vi "Meas Sequence Loop.vi"(8 "error in":errorcluster, 11 "meas session in":T1={"adc"={"niScope"={"channel cfg"=[], "sessions"=[], "multi cards"=FALSE, "channels"=0, "type"=enum."n/a", "memory [B/chn]"=0, "ext. clock [Hz]"=0.0, "samples count"=0, "use streaming"=FALSE, "proc setup"={"packet size [smpl]"=0, "current timeout [s]"=0.0, "blk2blk timeout [s]"=0.0, "event time"=timestamp(0 s since 1904-01-01), "temp sampl T [s]"=0.0, "data queue"=refnum, "stop notifier"=refnum, "proc ref"=refnum}, "sample width [B]"=0, "ranges [V]"=[], "trigger setup"={"coupling"=1, "level [V]"=0.0, "slope"=0, "mode"=enum."Immediate"}, "fs [Hz]"=0.0, "bitres [bit]"=0}, "3458A"={"channels"=[], "sync unit"={"VISA"="", "type"=enum."Picotest U6200A"}, "awg unit"={"type"=enum."Agilent 331xxA to 332xxA", "VISA"="", "enable 10MHz ref"=FALSE}, "sync mode"=enum."MASTER-SLAVE, MASTER clocked by TIMER", "streaming mode"=FALSE, "idn mode"=enum."Auto", "sampling mode"=enum."DCV", "Ts [s]"=0.0, "sample memory [B]"=0, "proc setup"={"channel id"=0, "packet size [smpl]"=0, "current timeout [s]"=0.0, "blk2blk timeout [s]"=0.0, "event time"=timestamp(0 s since 1904-01-01), "stop notifier"=refnum, "data queues"=[], "proc refs"=[], "bus semaphore"=refnum}, "sample size [B]"=0, "sample count"=0, "aux data"={"channel id"=0, "valid?"=[], "gain [V]"=[], "timestamp [s]"=[], "Ts [s]"=0.0, "abs timestamp"=timestamp(0 s since 1904-01-01), "t [deg C]"=[]}, "ranges [V]"=[], "aperture [s]"=0.0, "LEVEL trigger"={"edge"=enum."POS", "level [V]"=0.0, "coupling"=enum."DC"}, "trigger mode"=enum."AUTO", "measure temp.?"=FALSE, "disp mesages"=[], "shared bus?"=FALSE, "disable display?"=FALSE, "aper mode"=enum."Manual", "aper rules"=[]}, "dsdll"={"dsdll"={"dsdll path"=path "", "dsdll handle"=[], "output devices"=[], "capture devices"=[]}, "channels"=0, "device id"=0, "channel idns"=[], "proc setup"={"packet size [smpl]"=0, "current timeout [s]"=0.0, "blk2blk timeout [s]"=0.0, "event time"=timestamp(0 s since 1904-01-01), "data queue"=refnum, "stop notifier"=refnum, "proc ref"=refnum}, "samples count"=0, "fs [Hz]"=0.0}, "type"=enum."niScope", "channel idn str"=[], "aux instr idn str"=[], "modified?"=FALSE, "simadc"={"channels"=[], "range [V]"=0.0, "Ts step [s]"=0.0, "time [s]"=0.0, "fs [Hz]"=0.0, "count"=0, "smpl offset"=0, "set count"=0, "bit res"=0}, "force rst?"=FALSE, "exit mode"=enum."Immediate reset", "exit dly"=0.0, "exit tmr"=timestamp(0 s since 1904-01-01), "busy?"=FALSE, "accessed?"=FALSE, "QuADC session"={"channel cfg"=[], "sessions"=[], "multi cards"=FALSE, "channels"=0, "type"=enum."n/a", "memory [B/chn]"=0, "ext. clock [Hz]"=0.0, "samples count"=0, "use streaming"=FALSE, "proc setup"={"packet size [smpl]"=0, "current timeout [s]"=0.0, "blk2blk timeout [s]"=0.0, "event time"=timestamp(0 s since 1904-01-01), "temp sampl T [s]"=0.0, "data queue"=refnum, "stop notifier"=refnum, "proc ref"=refnum}, "sample width [B]"=0, "ranges [V]"=[], "trigger setup"={"coupling"=1, "level [V]"=0.0, "slope"=0, "mode"=enum."Immediate"}, "fs [Hz]"=0.0, "bitres [bit]"=0}}, "sequence"=[], "sequence setup"={"group setups"=[], "average cycles"=0, "range mode"=enum."Keep defaults", "fs mode"=enum."Frequency", "rng even"=0.0, "rng odd"=0.0, "folder"=path "", "name base"="", "meas id"=0, "settle [s]"=0.0}, "golpi"=refnum, "processing setup"={"mode"=enum."Raw", "call after avgs?"=FALSE, "calculate?"=FALSE, "raw mode"={"command"="", "result mode"=enum."Display console output (only Octave)", "res variable"=""}, "QWTB"={"QWTB path"=path "", "alg filter path"="", "alg ids"=[], "alg parameters"=[], "parsed parameters"=[], "selected alg id"="", "selected unc mode"=enum."None", "qwtb mcc"=100, "qwtb timeout"=90, "qwtb covg"=95.0, "qwtb ofs"=0, "qwtb lim data"=0, "multicore"={"jobs folder"=path "", "cores"=0, "max jobs"=0, "mode"=enum."Singlecore"}, "unc once?"=FALSE}}, "corrections"={"transducers"={"channels"=[], "last path"=path ""}, "digitizer"={"last path"=path "", "channel paths"=[], "channel idns"=[], "correction name"="", "channel names"=[], "folders to copy"=[], "channel valid"=[], "correction path"=path "", "correction rel path"="", "rel folders to copy"=[]}}, "assist cfg"={"P"=0, "Q"=0, "rel shift"=0.0, "ref freq"=0.0, "min fs"=0.0, "max fs tol"=0.0, "min int"=0.0, "max int"=0.0, "max err"=0.0, "max timeout"=0.0}} {"corrections"."transducers"."channels"."Phase index" min=1 step=1; "adc"."QuADC session"."trigger setup"."level [V]" format="%.2f"; "adc"."QuADC session"."trigger setup"."coupling" items=["AC"=0, "DC"=1, "HF Reject"=3, "LF Reject"=4, "AC Plus HF Reject"=1001]; "adc"."QuADC session"."channel cfg"."Clock fr. (Hz)" min=0.0 format="%#_9p"; "adc"."QuADC session"."channel cfg"."Number of JJ" min=1; "adc"."QuADC session"."channel cfg"."Range [Vpk]" min=0.0; "adc"."QuADC session"."channel cfg"."Channel" min=0; "adc"."3458A"."channels"."Range [Vpk]" min=0.0; "adc"."niScope"."trigger setup"."level [V]" format="%.2f"; "adc"."niScope"."trigger setup"."coupling" items=["AC"=0, "DC"=1, "HF Reject"=3, "LF Reject"=4, "AC Plus HF Reject"=1001]; "adc"."niScope"."channel cfg"."Range [Vpk]" min=0.0; "adc"."niScope"."channel cfg"."Channel" min=0}) -> (0 "error out":errorcluster, 3 "meas session out":T1={"adc"={"niScope"={"channel cfg"=[], "sessions"=[], "multi cards"=FALSE, "channels"=0, "type"=enum."n/a", "memory [B/chn]"=0, "ext. clock [Hz]"=0.0, "samples count"=0, "use streaming"=FALSE, "proc setup"={"packet size [smpl]"=0, "current timeout [s]"=0.0, "blk2blk timeout [s]"=0.0, "event time"=timestamp(0 s since 1904-01-01), "temp sampl T [s]"=0.0, "data queue"=refnum, "stop notifier"=refnum, "proc ref"=refnum}, "sample width [B]"=0, "ranges [V]"=[], "trigger setup"={"coupling"=1, "level [V]"=0.0, "slope"=0, "mode"=enum."Immediate"}, "fs [Hz]"=0.0, "bitres [bit]"=0}, "3458A"={"channels"=[], "sync unit"={"VISA"="", "type"=enum."Picotest U6200A"}, "awg unit"={"type"=enum."Agilent 331xxA to 332xxA", "VISA"="", "enable 10MHz ref"=FALSE}, "sync mode"=enum."MASTER-SLAVE, MASTER clocked by TIMER", "streaming mode"=FALSE, "idn mode"=enum."Auto", "sampling mode"=enum."DCV", "Ts [s]"=0.0, "sample memory [B]"=0, "proc setup"={"channel id"=0, "packet size [smpl]"=0, "current timeout [s]"=0.0, "blk2blk timeout [s]"=0.0, "event time"=timestamp(0 s since 1904-01-01), "stop notifier"=refnum, "data queues"=[], "proc refs"=[], "bus semaphore"=refnum}, "sample size [B]"=0, "sample count"=0, "aux data"={"channel id"=0, "valid?"=[], "gain [V]"=[], "timestamp [s]"=[], "Ts [s]"=0.0, "abs timestamp"=timestamp(0 s since 1904-01-01), "t [deg C]"=[]}, "ranges [V]"=[], "aperture [s]"=0.0, "LEVEL trigger"={"edge"=enum."POS", "level [V]"=0.0, "coupling"=enum."DC"}, "trigger mode"=enum."AUTO", "measure temp.?"=FALSE, "disp mesages"=[], "shared bus?"=FALSE, "disable display?"=FALSE, "aper mode"=enum."Manual", "aper rules"=[]}, "dsdll"={"dsdll"={"dsdll path"=path "", "dsdll handle"=[], "output devices"=[], "capture devices"=[]}, "channels"=0, "device id"=0, "channel idns"=[], "proc setup"={"packet size [smpl]"=0, "current timeout [s]"=0.0, "blk2blk timeout [s]"=0.0, "event time"=timestamp(0 s since 1904-01-01), "data queue"=refnum, "stop notifier"=refnum, "proc ref"=refnum}, "samples count"=0, "fs [Hz]"=0.0}, "type"=enum."niScope", "channel idn str"=[], "aux instr idn str"=[], "modified?"=FALSE, "simadc"={"channels"=[], "range [V]"=0.0, "Ts step [s]"=0.0, "time [s]"=0.0, "fs [Hz]"=0.0, "count"=0, "smpl offset"=0, "set count"=0, "bit res"=0}, "force rst?"=FALSE, "exit mode"=enum."Immediate reset", "exit dly"=0.0, "exit tmr"=timestamp(0 s since 1904-01-01), "busy?"=FALSE, "accessed?"=FALSE, "QuADC session"={"channel cfg"=[], "sessions"=[], "multi cards"=FALSE, "channels"=0, "type"=enum."n/a", "memory [B/chn]"=0, "ext. clock [Hz]"=0.0, "samples count"=0, "use streaming"=FALSE, "proc setup"={"packet size [smpl]"=0, "current timeout [s]"=0.0, "blk2blk timeout [s]"=0.0, "event time"=timestamp(0 s since 1904-01-01), "temp sampl T [s]"=0.0, "data queue"=refnum, "stop notifier"=refnum, "proc ref"=refnum}, "sample width [B]"=0, "ranges [V]"=[], "trigger setup"={"coupling"=1, "level [V]"=0.0, "slope"=0, "mode"=enum."Immediate"}, "fs [Hz]"=0.0, "bitres [bit]"=0}}, "sequence"=[], "sequence setup"={"group setups"=[], "average cycles"=0, "range mode"=enum."Keep defaults", "fs mode"=enum."Frequency", "rng even"=0.0, "rng odd"=0.0, "folder"=path "", "name base"="", "meas id"=0, "settle [s]"=0.0}, "golpi"=refnum, "processing setup"={"mode"=enum."Raw", "call after avgs?"=FALSE, "calculate?"=FALSE, "raw mode"={"command"="", "result mode"=enum."Display console output (only Octave)", "res variable"=""}, "QWTB"={"QWTB path"=path "", "alg filter path"="", "alg ids"=[], "alg parameters"=[], "parsed parameters"=[], "selected alg id"="", "selected unc mode"=enum."None", "qwtb mcc"=100, "qwtb timeout"=90, "qwtb covg"=95.0, "qwtb ofs"=0, "qwtb lim data"=0, "multicore"={"jobs folder"=path "", "cores"=0, "max jobs"=0, "mode"=enum."Singlecore"}, "unc once?"=FALSE}}, "corrections"={"transducers"={"channels"=[], "last path"=path ""}, "digitizer"={"last path"=path "", "channel paths"=[], "channel idns"=[], "correction name"="", "channel names"=[], "folders to copy"=[], "channel valid"=[], "correction path"=path "", "correction rel path"="", "rel folders to copy"=[]}}, "assist cfg"={"P"=0, "Q"=0, "rel shift"=0.0, "ref freq"=0.0, "min fs"=0.0, "max fs tol"=0.0, "min int"=0.0, "max int"=0.0, "max err"=0.0, "max timeout"=0.0}} {"corrections"."transducers"."channels"."Phase index" min=1 step=1; "adc"."QuADC session"."trigger setup"."level [V]" format="%.2f"; "adc"."QuADC session"."trigger setup"."coupling" items=["AC"=0, "DC"=1, "HF Reject"=3, "LF Reject"=4, "AC Plus HF Reject"=1001]; "adc"."QuADC session"."channel cfg"."Clock fr. (Hz)" min=0.0 format="%#_9p"; "adc"."QuADC session"."channel cfg"."Number of JJ" min=1; "adc"."QuADC session"."channel cfg"."Range [Vpk]" min=0.0; "adc"."QuADC session"."channel cfg"."Channel" min=0; "adc"."3458A"."channels"."Range [Vpk]" min=0.0; "adc"."niScope"."trigger setup"."level [V]" format="%.2f"; "adc"."niScope"."trigger setup"."coupling" items=["AC"=0, "DC"=1, "HF Reject"=3, "LF Reject"=4, "AC Plus HF Reject"=1001]; "adc"."niScope"."channel cfg"."Range [Vpk]" min=0.0; "adc"."niScope"."channel cfg"."Channel" min=0})   [LabVIEW 2013]
doc: "This VI initiates sampling of one record with current setup of ADC. It streams the sample data to MAT file of a given path (without extension). The VI also appends logged temperatures to the MAT file. It will return ADC auxiliary data which are valid only if flag 'valid?' in the cluster is True (that should happen all the time except when the sampling was aborted for whatever reason). The VI responds to global stop button called 'btn stop' - it will abort sampling when it is in True state."
uses:
  Meas Session.ctl
  adc/ADC Session.ctl
  drivers/niScope/niScope Session.ctl
  drivers/niScope/niScope Virtual Channel Config.ctl
  drivers/niScope/niScope Virtual Channel Mode.ctl
  drivers/niScope/niScope Virtual Channel Input Z.ctl
  drivers/niScope/niScope Virtual Channel Coupling.ctl
  drivers/niScope/niScope Type.ctl
  drivers/niScope/niScope Digitizing Process Options.ctl
  drivers/niScope/niScope Data Packet.ctl
  drivers/niScope/niScope Trigger Setup.ctl
  <instrlib>/niScope/Controls/niScope trigger coupling.ctl
  <instrlib>/niScope/Controls/niScope trigger slope.ctl
  drivers/DMM/3458A Digitizer Session.ctl
  drivers/DMM/3458A Virtual Channel Config.ctl
  drivers/Counter/Counter Session.ctl
  drivers/Counter/Counter Type.ctl
  drivers/AWG/AWG Session.ctl
  drivers/AWG/AWG Type.ctl
  drivers/DMM/3458A Sync Mode.ctl
  drivers/DMM/3458A Idn Mode.ctl
  drivers/DMM/3458A Digitizing Low Levels/Configure/Sampling Mode.ctl
  drivers/DMM/3458A Digitizing Process Options.ctl
  drivers/DMM/3458A Data Packet.ctl
  drivers/DMM/3458A Aux Record Data.ctl
  drivers/DMM/3458A Digitizing Low Levels/Configure/Level Setup.ctl
  drivers/DMM/3458A Digitizing Low Levels/Configure/First Sample Trigger.ctl
  drivers/DMM/3458A Aperture Selection Mode.ctl
  drivers/dsdll/DSDLL Session.ctl
  drivers/dsdll/dsdll.lvlibp/dsdll_instance.ctl
  drivers/dsdll/dsdll.lvlibp/dsdll_device_record.ctl
  drivers/dsdll/DSDLL Process Config.ctl
  drivers/dsdll/DSDLL Data Packet.ctl
  adc/ADC Type.ctl
  drivers/simulated_adc/SimAdc Config.ctl
  drivers/simulated_adc/SimAdc Channel Cfg.ctl
  adc/ADC On Close Action.ctl
  drivers/Quatsch_driver/QuADCDriver/QuADC Session.ctl
  drivers/Quatsch_driver/QuADCDriver/QuADC Virtual Channel Config.ctl
  drivers/Quatsch_driver/QuADCDriver/QuADC Virtual Channel Mode.ctl
  drivers/Quatsch_driver/QuADCDriver/QuADC Virtual Channel Input Z.ctl
  drivers/Quatsch_driver/QuADCDriver/QuADC Virtual Channel Coupling.ctl
  drivers/Quatsch_driver/QuADCDriver/QuADC Type.ctl
  drivers/Quatsch_driver/QuADCDriver/QuADC Digitizing Process Options.ctl
  drivers/Quatsch_driver/QuADCDriver/QuADC Data Packet.ctl
  drivers/Quatsch_driver/QuADCDriver/QuADC Trigger Setup.ctl
  Meas Sequence Item.ctl
  Meas Sampling Configuration.ctl
  adc/ADC Trig Config.ctl
  adc/ADC Trig Mode Source.ctl
  adc/ADC Trig Coupling.ctl
  adc/ADC Trig Slope.ctl
  processing/QWTB/Meas Proc QWTB Algorithm Parameter Data.ctl
  Meas Sequence Configuration.ctl
  Meas Range Mode.ctl
  Meas Sampling Rate Mode.ctl
  octave/golpi/mpc/golpi_session_ref.ctl
  octave/golpi/mpc/golpi_session.ctl
  octave/golpi/GOLPI Library.lvlibp/Public/GOLPI reference Type Def.ctl
  octave/golpi/GOLPI Library.lvlibp/LV Process source distribution/Pipe Handle.ctl
  processing/Meas Process Config.ctl
  processing/Meas Process Mode.ctl
  processing/Meas Process Raw Config.ctl
  processing/Meas Process Raw Result Mode.ctl
  processing/QWTB/Meas Proc QWTB Setup.ctl
  processing/QWTB/Meas Proc QWTB Uncertainty Mode.ctl
  processing/QWTB/Meas Proc QWTB Multicore Setup.ctl
  processing/QWTB/Meas Proc QWTB Multicore Type.ctl
  Corrections/Corr Setup.ctl
  Corrections/Corr Tranducer Item.ctl
  Corrections/Corr Digitizers.ctl
  Assist/Assist Panel Setup.ctl
  varilib/SGUI Assign Multiple Strings With Tags By Label.vi
  varilib/varilib.lvlib
  drivers/niScope/niScope Virtual Digitizer.lvlib
  drivers/DMM/3458A Virtual Digitizer.lvlib
  drivers/Counter/Counter.lvlib
  drivers/AWG/AWG.lvlib
  drivers/DMM/3458A Digitizing Low Levels/3458A Digitizing Low Levels.lvlib
  drivers/dsdll/dsdll.lvlibp
  drivers/dsdll/DSDLL Virtual Digitizer.lvlib
  octave/golpi/GOLPI Library.lvlibp/LV Process source distribution/LV Process library.lvlib
  octave/golpi/GOLPI Library.lvlibp
  octave/golpi/mpc/GOLPI Multi Process.lvlib
  drivers/Quatsch_driver/QuADCDriver/QuADC Virtual Digitizer.lvlib
panel:
  # "ADC:"
  # "IP Address"
  # "."
  # "."
  # "."
  # ":"
  # "ADC:"
  # "IP Address"
  # "."
  # "."
  # "."
  # ":"
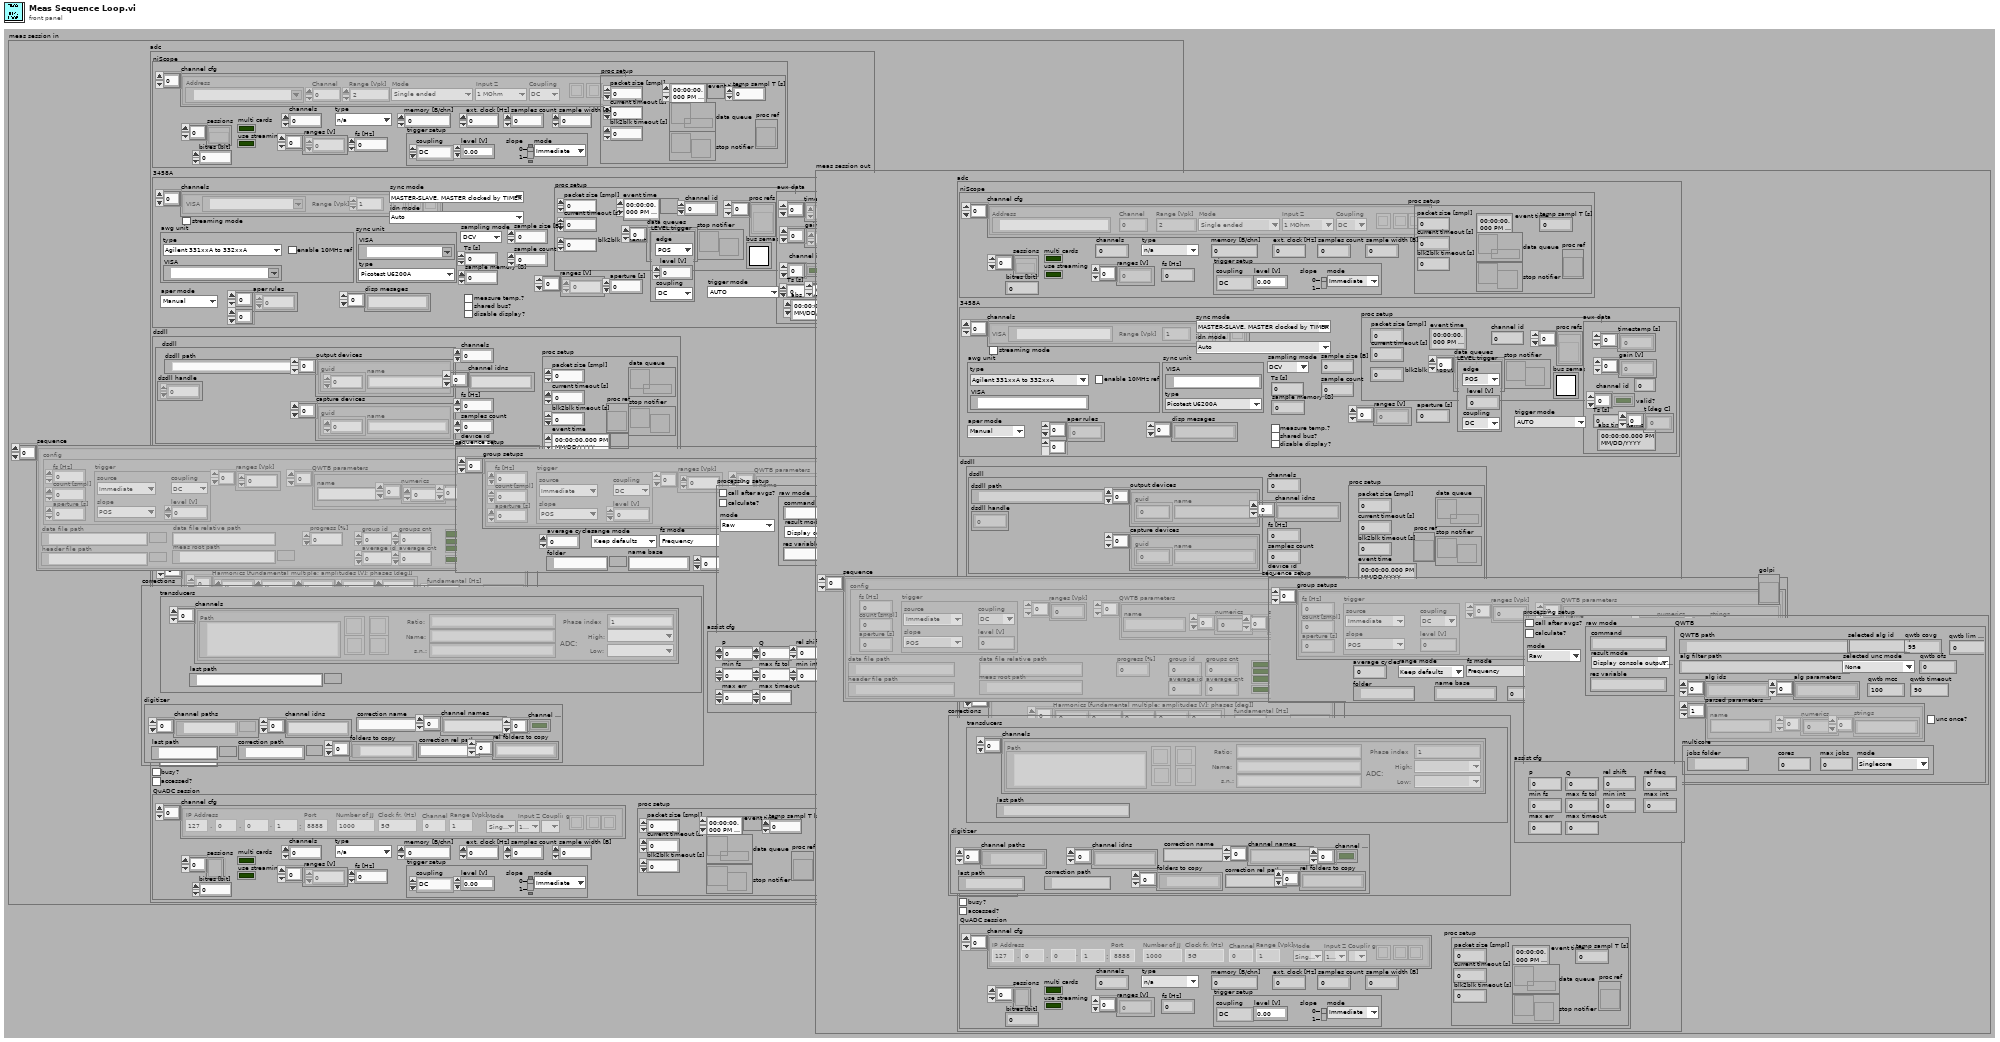
[diagram p1: front panel]
types:
  T1 = typedef "Meas Session.ctl" = cluster{"adc":T2, "sequence":T44[], "sequence setup":T51, "golpi":T54, "processing setup":T55, "corrections":T63, "assist cfg":T66}
  T2 = typedef "ADC Session.ctl" = cluster{"niScope":T3, "3458A":T13, "dsdll":T28, "type":T32, "channel idn str":string[], "aux instr idn str":string[], "modified?":bool, "simadc":T33, "force rst?":bool, "exit mode":T35, "exit dly":dbl, "exit tmr":timestamp, "busy?":bool, "accessed?":bool, "QuADC session":T36}
  T3 = typedef "niScope Virtual Digitizer.lvlib/niScope Session.ctl" = cluster{"channel cfg":T4[], "sessions":refnum<k20>[], "multi cards":bool, "channels":i32, "type":T8, "memory [B/chn]":i32, "ext. clock [Hz]":dbl, "samples count":i64, "use streaming":bool, "proc setup":T9, "sample width [B]":i32, "ranges [V]":dbl[], "trigger setup":T10, "fs [Hz]":dbl, "bitres [bit]":i32}
  T4 = typedef "niScope Virtual Digitizer.lvlib/niScope Virtual Channel Config.ctl" = cluster{"Address":refnum<k15>, "Channel":i32, "Mode":T5, "Input Z":T6, "Coupling":T7, "Range [Vpk]":dbl, "btn clr":bool, "btn up":bool, "btn down":bool}
  T5 = typedef "niScope Virtual Digitizer.lvlib/niScope Virtual Channel Mode.ctl" = enum16{"Single ended", "Unbal. differential", "Differential"}
  T6 = typedef "niScope Virtual Digitizer.lvlib/niScope Virtual Channel Input Z.ctl" = enum16{"1 MOhm", "50 Ohm"}
  T7 = typedef "niScope Virtual Digitizer.lvlib/niScope Virtual Channel Coupling.ctl" = enum16{"AC", "DC", "GND"}
  T8 = typedef "niScope Virtual Digitizer.lvlib/niScope Type.ctl" = enum16{"n/a", "5922"}
  T9 = typedef "niScope Virtual Digitizer.lvlib/niScope Digitizing Process Options.ctl" = cluster{"packet size [smpl]":i64, "current timeout [s]":dbl, "blk2blk timeout [s]":dbl, "event time":timestamp, "temp sampl T [s]":dbl, "data queue":refnum<queue>, "stop notifier":refnum<notifier>, "proc ref":refnum<vi>}
  T10 = typedef "niScope Virtual Digitizer.lvlib/niScope Trigger Setup.ctl" = cluster{"coupling":T11, "level [V]":dbl, "slope":T12, "mode":enum16{"Immediate", "External", "Level"}}
  T11 = typedef "niScope trigger coupling.ctl" = u16
  T12 = typedef "niScope trigger slope.ctl" = i32
  T13 = typedef "3458A Virtual Digitizer.lvlib/3458A Digitizer Session.ctl" = cluster{"channels":T14[], "sync unit":T15, "awg unit":T17, "sync mode":T19, "streaming mode":bool, "idn mode":T20, "sampling mode":T21, "Ts [s]":dbl, "sample memory [B]":i32, "proc setup":T22, "sample size [B]":i32, "sample count":i32, "aux data":T24, "ranges [V]":dbl[], "aperture [s]":dbl, "LEVEL trigger":T25, "trigger mode":T26, "measure temp.?":bool, "disp mesages":string[], "shared bus?":bool, "disable display?":bool, "aper mode":T27, "aper rules":dbl[][]}
  T14 = typedef "3458A Virtual Digitizer.lvlib/3458A Virtual Channel Config.ctl" = cluster{"VISA":refnum<visa-resource-name>, "Range [Vpk]":dbl, "btn clr":bool, "btn up":bool, "btn down":bool}
  T15 = typedef "Counter.lvlib/Counter Session.ctl" = cluster{"VISA":refnum<visa-resource-name>, "type":T16}
  T16 = typedef "Counter.lvlib/Counter Type.ctl" = enum16{"Picotest U6200A", "dummy"}
  T17 = typedef "AWG.lvlib/AWG Session.ctl" = cluster{"type":T18, "VISA":refnum<visa-resource-name>, "enable 10MHz ref":bool}
  T18 = typedef "AWG.lvlib/AWG Type.ctl" = enum16{"Agilent 331xxA to 332xxA", "Agilent 335xxA to 336xxA", "Tektronix AFG3101C", "dummy"}
  T19 = typedef "3458A Virtual Digitizer.lvlib/3458A Sync Mode.ctl" = enum16{"MASTER-SLAVE, MASTER clocked by TIMER", "MASTER-SLAVE, MASTER clocked by AWG", "ALL clocked by AWG", "MASTER-SLAVE, ALL clocked by TIMER", "ALL clocked by AWG with DFLL"}
  T20 = typedef "3458A Virtual Digitizer.lvlib/3458A Idn Mode.ctl" = enum16{"Auto", "Sequential (chn A, chn B, ...)", "From calibration string"}
  T21 = typedef "3458A Virtual Digitizer.lvlib/3458A Digitizing Low Levels.lvlib/Sampling Mode.ctl" = enum16{"DCV", "DSDC", "DSAC"}
  T22 = typedef "3458A Virtual Digitizer.lvlib/3458A Digitizing Process Options.ctl" = cluster{"channel id":i32, "packet size [smpl]":i32, "current timeout [s]":dbl, "blk2blk timeout [s]":dbl, "event time":timestamp, "stop notifier":refnum<notifier>, "data queues":refnum<queue>[], "proc refs":refnum<vi>[], "bus semaphore":T23}
  T23 = typedef "Semaphore RefNum" = refnum<k1>
  T24 = typedef "3458A Virtual Digitizer.lvlib/3458A Aux Record Data.ctl" = cluster{"channel id":i32, "valid?":bool[], "gain [V]":dbl[], "timestamp [s]":dbl[], "Ts [s]":dbl, "abs timestamp":timestamp, "t [deg C]":dbl[]}
  T25 = typedef "3458A Virtual Digitizer.lvlib/3458A Digitizing Low Levels.lvlib/Level Setup.ctl" = cluster{"edge":enum16{"POS", "NEG"}, "level [V]":dbl, "coupling":enum16{"DC", "AC"}}
  T26 = typedef "3458A Virtual Digitizer.lvlib/3458A Digitizing Low Levels.lvlib/First Sample Trigger.ctl" = enum16{"AUTO", "EXT", "SYN", "SGL", "HOLD", "LEVEL"}
  T27 = typedef "3458A Virtual Digitizer.lvlib/3458A Aperture Selection Mode.ctl" = enum16{"Manual", "Maximum", "Table"}
  T28 = typedef "DSDLL Virtual Digitizer.lvlib/DSDLL Session.ctl" = cluster{"dsdll":T29, "channels":i32, "device id":i32, "channel idns":string[], "proc setup":T31, "samples count":i32, "fs [Hz]":dbl}
  T29 = typedef "dsdll.lvlibp/dsdll_instance.ctl" = cluster{"dsdll path":path, "dsdll handle":u8[], "output devices":T30[], "capture devices":T30[]}
  T30 = typedef "dsdll.lvlibp/dsdll_device_record.ctl" = cluster{"guid":u8[], "name":string}
  T31 = typedef "DSDLL Virtual Digitizer.lvlib/DSDLL Process Config.ctl" = cluster{"packet size [smpl]":i32, "current timeout [s]":dbl, "blk2blk timeout [s]":dbl, "event time":timestamp, "data queue":refnum<queue>, "stop notifier":refnum<notifier>, "proc ref":refnum<vi>}
  T32 = typedef "ADC Type.ctl" = enum16{"niScope", "3458A", "DirectSound DLL", "dummy", "QuADC"}
  T33 = typedef "SimAdc Config.ctl" = cluster{"channels":T34[], "range [V]":dbl, "Ts step [s]":dbl, "time [s]":dbl, "fs [Hz]":dbl, "count":i64, "smpl offset":i64, "set count":i64, "bit res":i32}
  T34 = typedef "SimAdc Channel Cfg.ctl" = cluster{"harmonics":dbl[][], "btn clear":bool, "noise":dbl, "fundamental [Hz]":dbl}
  T35 = typedef "ADC On Close Action.ctl" = enum16{"Immediate reset", "Delayed reset"}
  T36 = typedef "QuADC Virtual Digitizer.lvlib/QuADC Session.ctl" = cluster{"channel cfg":T37[], "sessions":refnum<k5>[], "multi cards":bool, "channels":i32, "type":T41, "memory [B/chn]":i32, "ext. clock [Hz]":dbl, "samples count":i64, "use streaming":bool, "proc setup":T42, "sample width [B]":i32, "ranges [V]":dbl[], "trigger setup":T43, "fs [Hz]":dbl, "bitres [bit]":i32}
  T37 = typedef "QuADC Virtual Digitizer.lvlib/QuADC Virtual Channel Config.ctl" = cluster{"Channel":i32, "Mode":T38, "Input Z":T39, "Coupling":T40, "Range [Vpk]":dbl, "btn clr":bool, "btn up":bool, "btn down":bool, "IP address A":u8, "IP address B":u8, "IP address C":u8, "IP address D":u8, "Port":u16, "Number of JJ":u32, "Clock fr. (Hz)":dbl}
  T38 = typedef "QuADC Virtual Digitizer.lvlib/QuADC Virtual Channel Mode.ctl" = enum16{"Single ended", "Unbal. differential", "Differential"}
  T39 = typedef "QuADC Virtual Digitizer.lvlib/QuADC Virtual Channel Input Z.ctl" = enum16{"1 MOhm", "50 Ohm"}
  T40 = typedef "QuADC Virtual Digitizer.lvlib/QuADC Virtual Channel Coupling.ctl" = enum16{"AC", "DC", "GND"}
  T41 = typedef "QuADC Virtual Digitizer.lvlib/QuADC Type.ctl" = enum16{"n/a", "v1"}
  T42 = typedef "QuADC Virtual Digitizer.lvlib/QuADC Digitizing Process Options.ctl" = cluster{"packet size [smpl]":i64, "current timeout [s]":dbl, "blk2blk timeout [s]":dbl, "event time":timestamp, "temp sampl T [s]":dbl, "data queue":refnum<queue>, "stop notifier":refnum<notifier>, "proc ref":refnum<vi>}
  T43 = typedef "QuADC Virtual Digitizer.lvlib/QuADC Trigger Setup.ctl" = cluster{"coupling":T11, "level [V]":dbl, "slope":T12, "mode":enum16{"Immediate", "External", "Level"}}
  T44 = typedef "Meas Sequence Item.ctl" = cluster{"config":T45, "data file path":path, "header file path":path, "group id":i32, "average id":i32, "group done?":bool, "adc modified?":bool, "source modified?":bool, "progress [%]":dbl, "groups cnt":i32, "average cnt":i32, "data file relative path":string, "meas root path":path, "calculate?":bool}
  T45 = typedef "Meas Sampling Configuration.ctl" = cluster{"fs [Hz]":dbl, "count [smpl]":i64, "aperture [s]":dbl, "trigger":T46, "ranges [Vpk]":dbl[], "QWTB parameters":T50[]}
  T46 = typedef "ADC Trig Config.ctl" = cluster{"source":T47, "level [V]":dbl, "coupling":T48, "slope":T49}
  T47 = typedef "ADC Trig Mode Source.ctl" = enum16{"Immediate", "External", "Level"}
  T48 = typedef "ADC Trig Coupling.ctl" = enum16{"DC", "AC"}
  T49 = typedef "ADC Trig Slope.ctl" = enum16{"POS", "NEG"}
  T50 = typedef "Meas Proc QWTB Algorithm Parameter Data.ctl" = cluster{"name":string, "numerics":dbl[], "strings":string[]}
  T51 = typedef "Meas Sequence Configuration.ctl" = cluster{"group setups":T45[], "average cycles":i32, "range mode":T52, "fs mode":T53, "rng even":dbl, "rng odd":dbl, "folder":path, "name base":string, "meas id":i32, "settle [s]":dbl}
  T52 = typedef "Meas Range Mode.ctl" = enum16{"Keep defaults", "Set All channels", "Set Odd and Even channels"}
  T53 = typedef "Meas Sampling Rate Mode.ctl" = enum16{"Frequency", "Period"}
  T54 = typedef "GOLPI Multi Process.lvlib/golpi_session_ref.ctl" = refnum<vi>
  T55 = typedef "Meas Process Config.ctl" = cluster{"mode":T56, "call after avgs?":bool, "calculate?":bool, "raw mode":T57, "QWTB":T59}
  T56 = typedef "Meas Process Mode.ctl" = enum16{"Raw", "QWTB"}
  T57 = typedef "Meas Process Raw Config.ctl" = cluster{"command":string, "result mode":T58, "res variable":string}
  T58 = typedef "Meas Process Raw Result Mode.ctl" = enum16{"Display console output (only Octave)", "Display string variable", "Display result file %respath%"}
  T59 = typedef "Meas Proc QWTB Setup.ctl" = cluster{"QWTB path":path, "alg filter path":string, "alg ids":string[], "alg parameters":string[], "parsed parameters":T50[], "selected alg id":string, "selected unc mode":T60, "qwtb mcc":i32, "qwtb timeout":i32, "qwtb covg":dbl, "qwtb ofs":i64, "qwtb lim data":i64, "multicore":T61, "unc once?":bool}
  T60 = typedef "Meas Proc QWTB Uncertainty Mode.ctl" = enum16{"None", "GUF", "Monte Carlo"}
  T61 = typedef "Meas Proc QWTB Multicore Setup.ctl" = cluster{"jobs folder":path, "cores":i32, "max jobs":i32, "mode":T62}
  T62 = typedef "Meas Proc QWTB Multicore Type.ctl" = enum16{"Singlecore", "Multicore", "Multistation"}
  T63 = typedef "Corr Setup.ctl" = cluster{"transducers":cluster{"channels":T64[], "last path":path}, "digitizer":T65}
  T64 = typedef "Corr Tranducer Item.ctl" = cluster{"Path":path, "Ratio:":string, "Name:":string, "btn rem":bool, "btn up":bool, "btn down":bool, "s.n.:":string, "btn open":bool, "ratio o/i":dbl, "chn hi":u16, "chn lo":u16, "Phase index":i32}
  T65 = typedef "Corr Digitizers.ctl" = cluster{"last path":path, "channel paths":path[], "channel idns":string[], "correction name":string, "channel names":string[], "folders to copy":path[], "channel valid":bool[], "correction path":path, "correction rel path":string, "rel folders to copy":string[]}
  T66 = typedef "Assist Panel Setup.ctl" = cluster{"P":i32, "Q":i32, "rel shift":dbl, "ref freq":dbl, "min fs":dbl, "max fs tol":dbl, "min int":dbl, "max int":dbl, "max err":dbl, "max timeout":dbl}
  T67 = typedef "ADC Aux Data.ctl" = cluster{"offset [V]":dbl[], "gain [V]":dbl[], "time stamp [s]":dbl[], "increment [s]":dbl, "T smpl":i64[], "T [deg C]":dbl[][], "valid?":bool, "abs timestamp":timestamp}
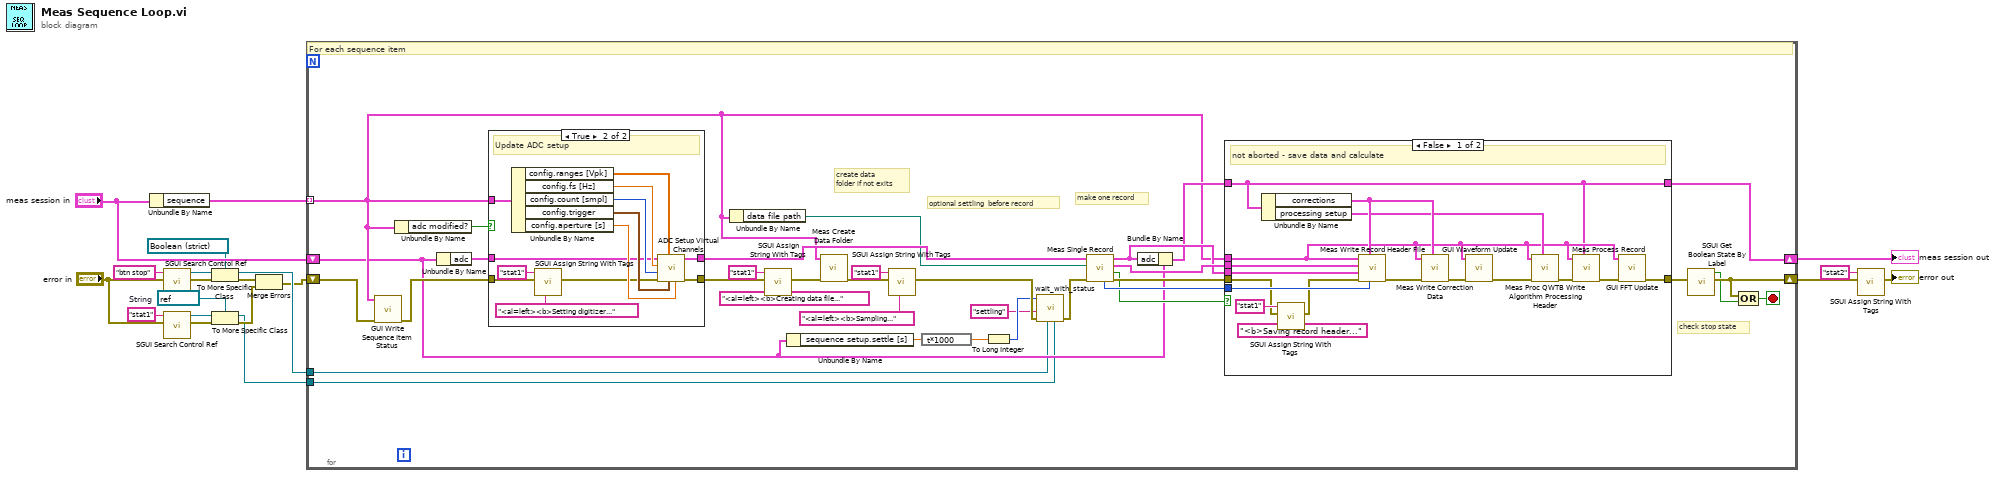
[diagram p0: block diagram]
diagram:
  w3 = refnum<vi> refnum  # String
  n1 = Unbundle By Name("meas session in") -> ("sequence"=w19:T44[])
  n2 = call "SGUI Search Control Ref.vi"("error in"="error in", "control label (empty)"="btn stop") -> ("error out"=w13:errorcluster, "control ref out"=w11:refnum<vi>)  [unwired: 7 in, 1 out]
  n3 = call "SGUI Search Control Ref.vi"("error in"="error in", "control label (empty)"="stat1") -> ("error out"=w9:errorcluster, "control ref out"=w5:refnum<vi>)  [unwired: 7 in, 1 out]
  n4 = To More Specific Class(target class=refnum<vi> refnum ("Boolean"), reference=w11, error in=w13) -> (specific class reference=w12:refnum<vi>, error out=w8:errorcluster)
  n5 = To More Specific Class(target class=w3, reference=w5, error in=w9) -> (specific class reference=w4:refnum<vi>, error out=w7:errorcluster)
  n6 = Merge Errors(w8, w7) -> (w6:errorcluster)
  n7 = for {
    tunnel: w19 -> [w31] mode=indexing
    shift-right: [w45] -> w18
    shift-left: w6 -> [w30]
    shift-right: [w32] -> w20
    shift-left: "meas session in" -> [w27]
    tunnel: w12 -> [w23]
    tunnel: w4 -> [w22]
    stop <- w46 stop-if-true
    # "optional settling  before record"
    # "create data\nfolder if not exits"
    # "check stop state"
    # "make one record"
    # "For each sequence item"
    n8 = call "GUI Write Sequence Item Status.vi"("error in"=w30, "sequence item"=w31) -> ("error out"=w35:errorcluster)  [unwired: 8 in, 1 out]
    n9 = Unbundle By Name(w31) -> ("adc modified?"=w53:bool)
    n10 = Unbundle By Name(w27) -> ("adc"=w54:T2)
    n11 = case shown="True" w53 {
      tunnel: w35 -> [w74 w79]
      tunnel: w31 -> [_ w83]
      tunnel: w54 -> [w75 w82]
      tunnel: [w74 w81] -> w42
      tunnel: [w75 w80] -> w48
      frame False {
      }
      frame True {
        # "Update ADC setup"
        n12 = Unbundle By Name(w83) -> ("config.ranges [Vpk]"=w88:dbl[], "config.fs [Hz]"=w87:dbl, "config.count [smpl]"=w86:i64, "config.trigger"=w85:T46, "config.aperture [s]"=w84:dbl)
        n13 = call-poly "SGUI Assign String With Tags.vi"("error in"=w79, "label(s) (empty)"="stat1", "string (empty)"="<al=left><b>Setting digitizer...") -> ("error out"=w78:errorcluster)  [unwired: 7 in, 1 out]
        n14 = call "ADC Setup Virtual Channels.vi"("apperture [s] (1.4 us)"=w84, "trigger (immediate)"=w85, "voltage ranges [Vpk] (empty: use global default)"=w88, "error in"=w78, "samples count (100)"=w86, "fs [Hz] (50k)"=w87, "adc session in"=w82) -> ("error out"=w81:errorcluster, "adc session out"=w80:T2)  [unwired: 3 in]
      }
    }
    n15 = Unbundle By Name(w31) -> ("data file path"=w34:path)
    n16 = call-poly "SGUI Assign String With Tags.vi"("error in"=w42, "label(s) (empty)"="stat1", "string (empty)"="<al=left><b>Creating data file...") -> ("error out"=w41:errorcluster)  [unwired: 7 in, 1 out]
    n17 = Unbundle By Name(w27) -> ("sequence setup.settle [s]"=w26:dbl)
    n18 = call "Meas Create Data Folder.vi"("error in"=w41, "sequence item"=w31) -> ("error out"=w38:errorcluster)  [unwired: 9 in]
    n19 = call-poly "SGUI Assign String With Tags.vi"("error in"=w38, "label(s) (empty)"="stat1", "string (empty)"="<al=left><b>Sampling...") -> ("error out"=w29:errorcluster)  [unwired: 7 in, 1 out]
    n20 = expression code="t*1000"(w26) -> (w25:dbl)
    n21 = To Long Integer(number=w25) -> (32bit integer=w24:i32)
    n22 = call "wait_with_status.vi"("stat ref"=w22, "stop ref"=w23, "error in"=w29, "comment"="settling", "ms to wait"=w24) -> ("error out"=w28:errorcluster)  [unwired: 6 in]
    n23 = call "Meas Single Record.vi"("error in"=w28, "binary data file path (no ext.)"=w34, "adc session in"=w48) -> ("error out"=w52:errorcluster, "aborted?"=w47:bool, "aux data"=w51:T67, "adc session out"=w50:T2, "acquired samples per channel"=w49:i64)  [unwired: 4 in]
    n24 = Bundle By Name(cluster=w27, "adc"=w50) -> (w33:T1)
    n25 = case shown="False" w47 {
      tunnel: w52 -> [w67 w73]
      tunnel: w51 -> [w71 _]
      tunnel: [w57 w73] -> w43
      tunnel: w31 -> [w56 _]
      tunnel: w50 -> [w70 _]
      tunnel: w49 -> [w69 _]
      tunnel: [w55 w72] -> w32
      tunnel: w33 -> [w55 w72]
      frame False {
        # "not aborted - save data and calculate"
        n26 = Unbundle By Name(w55) -> ("corrections"=w63:T63, "processing setup"=w59:T55)
        n27 = call-poly "SGUI Assign String With Tags.vi"("error in"=w67, "label(s) (empty)"="stat1", "string (empty)"="<b>Saving record header...") -> ("error out"=w66:errorcluster)  [unwired: 7 in, 1 out]
        n28 = call "Meas Write Record Header File.vi"("samples count"=w69, "corrections"=w63, "error in"=w66, "adc session"=w70, "aux data"=w71, "sequence item"=w56) -> ("error out"=w64:errorcluster)  [unwired: 5 in]
        n29 = call "Meas Write Correction Data.vi"("corrections"=w63, "error in"=w64, "sequence item"=w56) -> ("error out"=w62:errorcluster)  [unwired: 8 in]
        n30 = call "GUI Waveform Update.vi"("error in"=w62, "sequence item"=w56) -> ("error out"=w61:errorcluster)  [unwired: 9 in]
        n31 = call "Meas Proc QWTB Write Algorithm Processing Header.vi"("processing setup"=w59, "error in"=w61, "sequence item"=w56) -> ("error out"=w60:errorcluster)  [unwired: 8 in]
        n32 = call "Meas Process Record.vi"("session"=w55, "error in"=w60, "sequence item"=w56) -> ("error out"=w58:errorcluster)  [unwired: 8 in]
        n33 = call "GUI FFT Update.vi"("error in"=w58, "sequence item"=w56) -> ("error out"=w57:errorcluster)  [unwired: 9 in]
      }
      frame True {
        # "aborted"
      }
    }
    n34 = call "SGUI Get Boolean State By Label.vi"("error in"=w43) -> ("error out"=w45:errorcluster, "binary state out"=w44:bool)  [unwired: 8 in, 1 out]
    n35 = Compound Arithmetic op=OR(w45, w44) -> (w46:bool)
  }
  "meas session out" <- w20
  n36 = call-poly "SGUI Assign String With Tags.vi"("error in"=w18, "label(s) (empty)"="stat2") -> ("error out"=→"error out":errorcluster)  [unwired: 8 in, 1 out]
